vi "Set Ramp.vi"(8 "error in (no error)":errorcluster, 10 "VoltageRampRate (V/s)":dbl, 11 "DriveMotors in":refnum<class "DriveMotors.lvclass">) -> (0 "error out":errorcluster, 3 "DriveMotors out":refnum<class "DriveMotors.lvclass">)   [LabVIEW 2013, in "DriveMotors.lvclass"]
uses:
  DriveMotors.lvclass
  DriveMotors.lvclass/DriveMotors.ctl
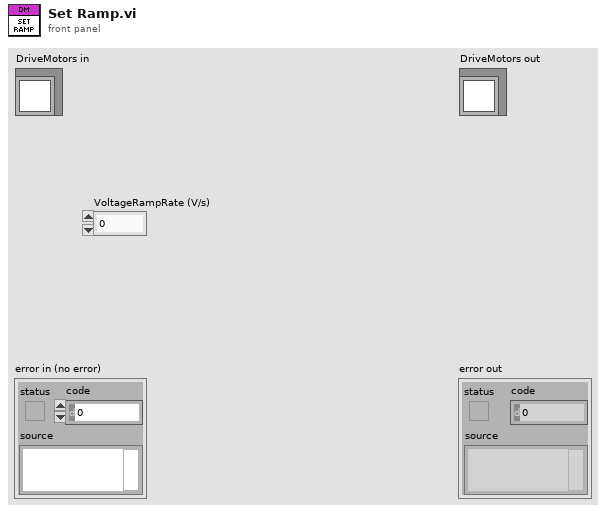
[diagram p1: front panel]
types:
  T1 = typedef "WPI_MotorControlDeviceRef.ctl" = cluster{"DeviceStatus":errorcluster, "Type":enum16{"PWM", "CAN"}, "PWM":cluster{"Digital Module":T2, "PWM Channel":T3, "DeadBand":T4}, "CAN":cluster{"Device Number":u8, "Control Mode":T5, "Semaphore":T6, "Max Vout":dbl}, "Invert":bool, "TransformRef":T7, "InvTransformRef":T7}
  T2 = typedef "FPGA_TypedefDigitalModule.ctl" = enum16{"Digital Module 1", "Digital Module 2"}
  T3 = typedef "FPGA_DIOPWMChannel.ctl" = enum8{"PWM 1", "PWM 2", "PWM 3", "PWM 4", "PWM 5", "PWM 6", "PWM 7", "PWM 8", "PWM 9", "PWM 10", "Invalid"}
  T4 = typedef "WPI_PWMDeadband.ctl" = cluster{"Name":string, "maxPositivePwm":i32, "minPositivePwm":i32, "centerPwm":i32, "maxNegativePwm":i32, "minNegativePwm":i32, "angularRange":u16}
  T5 = typedef "WPI_CANJaguar_ControlMode.ctl" = enum8{"Percent VBus", "Current", "Speed", "Position", "Voltage"}
  T6 = typedef "Semaphore RefNum" = refnum<k1>
  T7 = typedef "WPI_PWMTransform_ConPane.ctl" = refnum<vi>
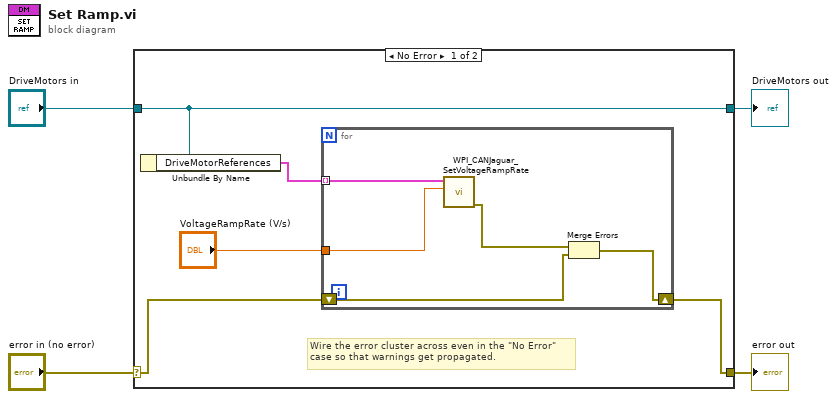
[diagram p0: block diagram]
diagram:
  n1 = case shown="No Error" "error in (no error)" {
    selector: "error in (no error)" -> [w6 w16]
    tunnel: [w5 w16] -> w3
    tunnel: [w9 w15] -> w1
    tunnel: "DriveMotors in" -> [w9 w15]
    frame No Error {
      # "Wire the error cluster across even in the \"No Error\"\ncase so that warnings get propagated."
      n2 = Unbundle By Name(w9) -> ("DriveMotorReferences"=w8:T1[])
      n3 = for {
        tunnel: w8 -> [w14] mode=indexing
        tunnel: "VoltageRampRate (V/s)" -> [w13]
        shift-right: [w10] -> w5
        shift-left: w6 -> [w11]
        n4 = call <vilib>:"WPI_CANJaguar_SetVoltageRampRate.vi"("VoltageRampRate (V/s)"=w13, "CAN Jaguar Ref"=w14) -> ("error out"=w12:errorcluster)  [unwired: 8 in, 1 out]
        n5 = Merge Errors(w12, w11) -> (w10:errorcluster)
      }
    }
    frame Error {
    }
  }
  "error out" <- w3
  "DriveMotors out" <- w1
